vi "WriteInLogger.vi"(8 "错误输入":errorcluster, 9 "LoggerData":string, 10 "refnum":refnum<file>) -> (0 "错误输出":errorcluster)   [LabVIEW 2019, in "Logger.lvclass"]
uses:
  <userlib>/Logger/Logger.lvclass
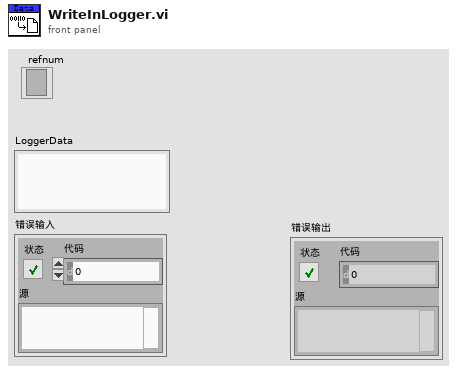
[diagram p1: front panel]
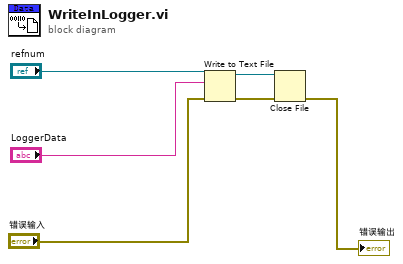
[diagram p0: block diagram]
diagram:
  n1 = Write to Text File(file (use dialog)="refnum", text="LoggerData", error in="错误输入") -> (refnum out=w3:refnum<file>, error out=w2:errorcluster)  [unwired: 1 in, 1 out]
  n2 = Close File(refnum=w3, error in=w2) -> (error out=→"错误输出":errorcluster)  [unwired: 1 out]
